vi "QPlus_Lockin_Analyzer.vi"() -> ()   [LabVIEW 2016]
uses:
  <instrlib>/Stanford Research 830/Public/Data/Read (1 Parameter).vi
  <vilib>/Utility/file.llb/Write Delimited Spreadsheet (DBL).vi
  <instrlib>/Stanford Research 830/Stanford Research 830.lvlib
panel:
  out "FWHM":dbl
  out "Quality Factor":dbl
  out "Integrated Signal":cluster{"Y":dbl[], "Y":dbl[]}[](graph)
  out "Resonance Frequency":dbl
  in  "VISA resource name":refnum<visa-resource-name>
  in  "Sensitivity (26: 1 V/uA)":i8(ring)=26 items=["Auto Gain"=-1, "2 nV/fA"=0, "5 nV/fA"=1, "10 nV/fA"=2, "20 nV/fA"=3, "50 nV/fA"=4, "100 nV/fA"=5, "200 nV/fA"=6, "500 nV/fA"=7, "1 uV/pA"=8, "2 uV/pA"=9, "5 uV/pA"=10, "10 uV/pA"=11, "20 uV/pA"=12, "50 uV/pA"=13, "100 uV/pA"=14, "200 uV/pA"=15, "500 uV/pA"=16, "1 mV/nA"=17, "2 mV/nA"=18, "5 mV/nA"=19, "10 mV/nA"=20, "20 mV/nA"=21, "50 mV/nA"=22, "100 mV/nA"=23, "200 mV/nA"=24, "500 mV/mA"=25, "1 V/uA"=26]
  in  "Time Constant (8: 100ms)":u16(ring)=8 items=["10 us", "30 us", "100 us", "300 us", "1 ms", "3 ms", "10 ms", "30 ms", "100 ms", "300 ms", "1 s", "3 s", "10 s", "30 s", "100 s", "300 s", "1 ks", "3 ks", "10 ks", "30 ks"]
  out "Raw Signal":cluster{"Y":dbl[], "Y":dbl[]}[](graph)
  in  "Save File Name":path=path "G:/UCB/Instruments/tip making/Qplus AFM tip making/qplus test/Caihong/CJ39.xlsx" caption="Filename"
  in  "Time Between Points (sec)":dbl=0.05 format="%#_1f"
  in  "Sine Output Amplitude (1 V)":dbl=1.0
  in  "Starting Frequency (Hz)":i32=32000
  in  "Final Frequency (Hz)":i32=33000
  in  "Step Size (Hz)":i32=10
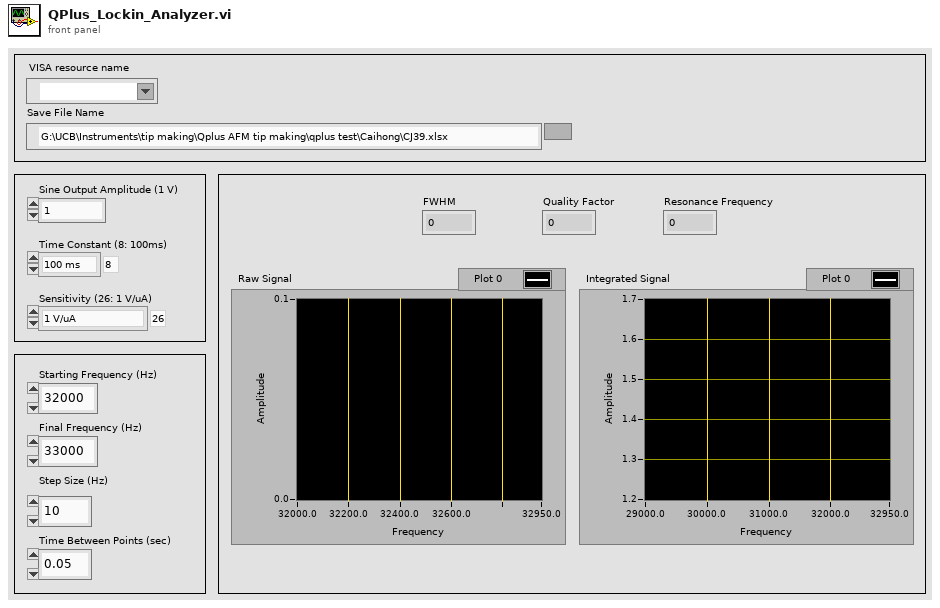
[diagram p1: front panel]
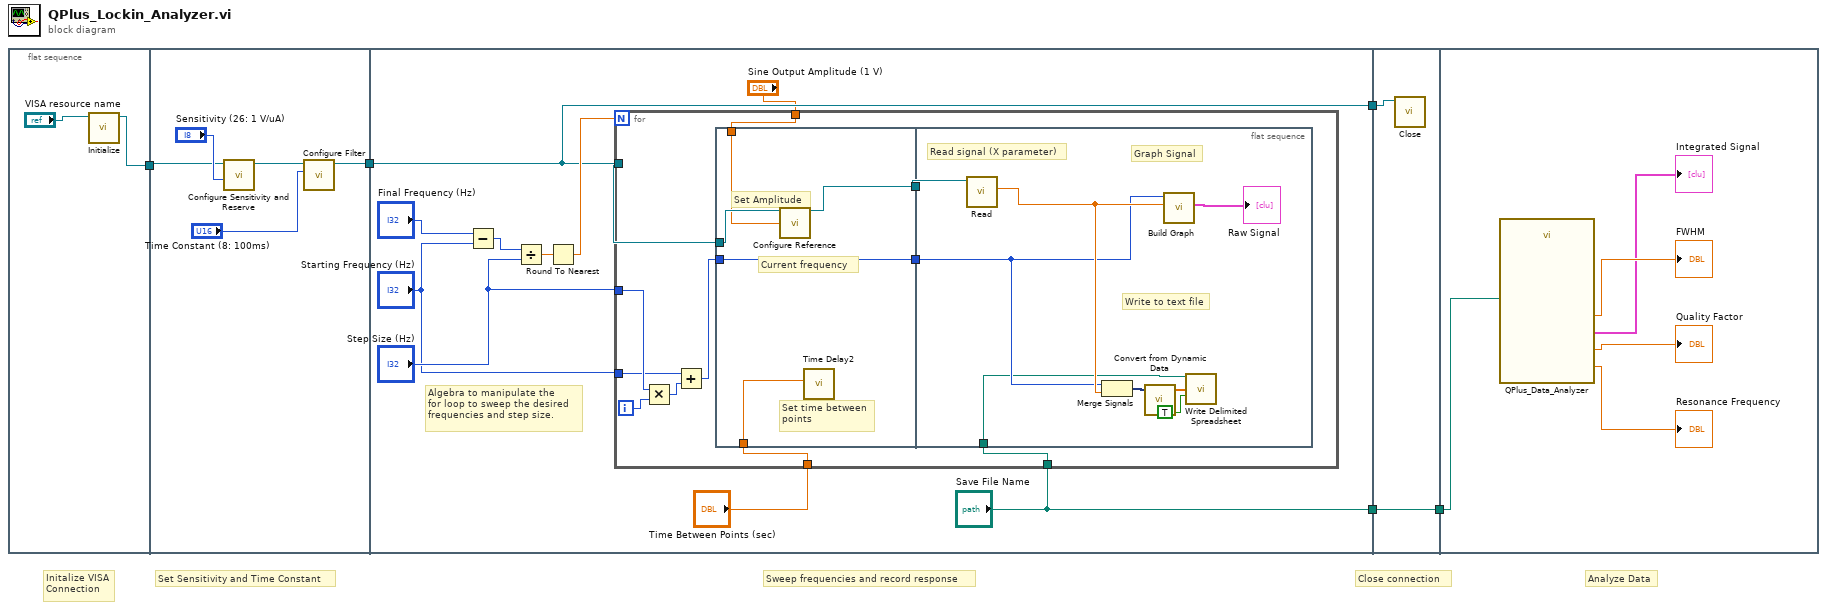
[diagram p0: block diagram]
diagram:
  # "Analyze Data"
  # "Close connection"
  # "Sweep frequencies and record response"
  # "Set Sensitivity and Time Constant"
  # "Initalize VISA\nConnection"
  n1 = flat-sequence {
    tunnel: [w6] -> w4
    tunnel: [w9] -> w5
    tunnel: w4 -> [w8]
    tunnel: w5 -> [w16]
    tunnel: [w16] -> w3
    tunnel: ["Save File Name"] -> w2
    tunnel: w3 -> [w48]
    tunnel: w2 -> [w47]
    tunnel: [w47] -> w1
    tunnel: w1 -> [w53]
    frame #0 {
      n2 = call <instrlib>:"Initialize.vi"("VISA resource name"="VISA resource name") -> ("VISA resource name out"=w6:refnum<visa-resource-name>)  [unwired: 9 in, 1 out]
    }
    frame #1 {
      n3 = call <instrlib>:"Configure Sensitivity and Reserve.vi"("Sensitivity (-1: Auto gain)"="Sensitivity (26: 1 V/uA)", "VISA resource name"=w8) -> ("VISA resource name out"=w11:refnum<visa-resource-name>)  [unwired: 8 in, 1 out]
      n4 = call <instrlib>:"Configure Filter.vi"("Time Constant (8: 100ms)"="Time Constant (8: 100ms)", "VISA resource name"=w11) -> ("VISA resource name out"=w9:refnum<visa-resource-name>)  [unwired: 8 in, 1 out]
    }
    frame #2 {
      # "Algebra to manipulate the\nfor loop to sweep the desired\nfrequencies and step size."
      n5 = Subtract(x="Final Frequency (Hz)", y="Starting Frequency (Hz)") -> (x-y=w21:i32)
      n6 = Divide(x=w21, y="Step Size (Hz)") -> (x/y=w20:dbl)
      n7 = Round To Nearest(number=w20) -> (nearest integer value=w17:dbl)
      n8 = for {
        N: w17 -> [_]
        tunnel: "Step Size (Hz)" -> [w32]
        tunnel: "Starting Frequency (Hz)" -> [w30]
        tunnel: w16 -> [w26]
        tunnel: "Time Between Points (sec)" -> [w25]
        tunnel: "Save File Name" -> [w24]
        tunnel: "Sine Output Amplitude (1 V)" -> [w23]
        i -> [w33]
        n9 = Multiply(x=w32, y=w33) -> (x*y=w31:i32)
        n10 = Add(x=w30, y=w31) -> (x+y=w27:i32)
        n11 = flat-sequence {
          tunnel: [w38] -> w29
          tunnel: [w37] -> w28
          tunnel: w27 -> [w37]
          tunnel: w26 -> [w36]
          tunnel: w25 -> [w35]
          tunnel: w23 -> [w34]
          tunnel: w29 -> [w41]
          tunnel: w28 -> [w40]
          tunnel: w24 -> [w39]
          frame #0 {
            # "Set Amplitude"
            # "Current frequency"
            # "Set time between\npoints"
            n12 = call <instrlib>:"Configure Reference.vi"("VISA resource name"=w36, "Sine Output Amplitude (1 V)"=w34) -> ("VISA resource name out"=w38:refnum<visa-resource-name>)  [unwired: 12 in, 1 out]
            n13 = call "Time Delay2"("Delay Time (s)"=w35) -> ()  [unwired: 10 in, 1 out]
          }
          frame #1 {
            # "Read signal (X parameter)"
            # "Graph Signal"
            # "Write to text file"
            n14 = call-poly <instrlib>:"Read.vi"("VISA resource name"=w41) -> ("Measurement"=w45:dbl)  [unwired: 8 in, 2 out]
            n15 = Merge Signals(w40, w45) -> (w43:dynamicdata)
            n16 = call "Convert from Dynamic Data"("Dynamic Data Type"=w43) -> ("Array"=w42:dbl[])  [unwired: 3 in]
            n17 = call "Build Graph"("Y Input"=w45, "X Input"=w40) -> ("XY Graph"=→"Raw Signal":cluster{"Y":dbl[], "Y":dbl[]}[])  [unwired: 3 in, 6 out]
            n18 = call-poly <vilib>:"Write Delimited Spreadsheet.vi"("file path (dialog if empty)"=w39, "1D data"=w42, "append to file? (new file:F)"=TRUE) -> ()  [unwired: 11 in, 2 out]
          }
        }
      }
    }
    frame #3 {
      n19 = call <instrlib>:"Close.vi"("VISA resource name"=w48) -> ()  [unwired: 10 in, 1 out]
    }
    frame #4 {
      n20 = call "QPlus_Data_Analyzer.vi"("File Path"=w53) -> ("Resonance Frequency"=→"Resonance Frequency":dbl, "Quality Factor"=→"Quality Factor":dbl, "FWHM"=→"FWHM":dbl, "Integrated Signal"=→"Integrated Signal":cluster{"Y":dbl[], "Y":dbl[]}[])  [unwired: 7 in]
    }
  }
